vi "Project documentation.vi"(8 "error in":errorcluster, 10 "Theme":bool, 11 "Project in":refnum<vi>) -> (0 "error out":errorcluster)   [LabVIEW 2019, in "Panther Dashboard.lvlib"]
uses:
  Panther Dashboard.lvlib
panel:
  in  "Cancel":bool
  in  "Save":bool
  in  "Project Description":string
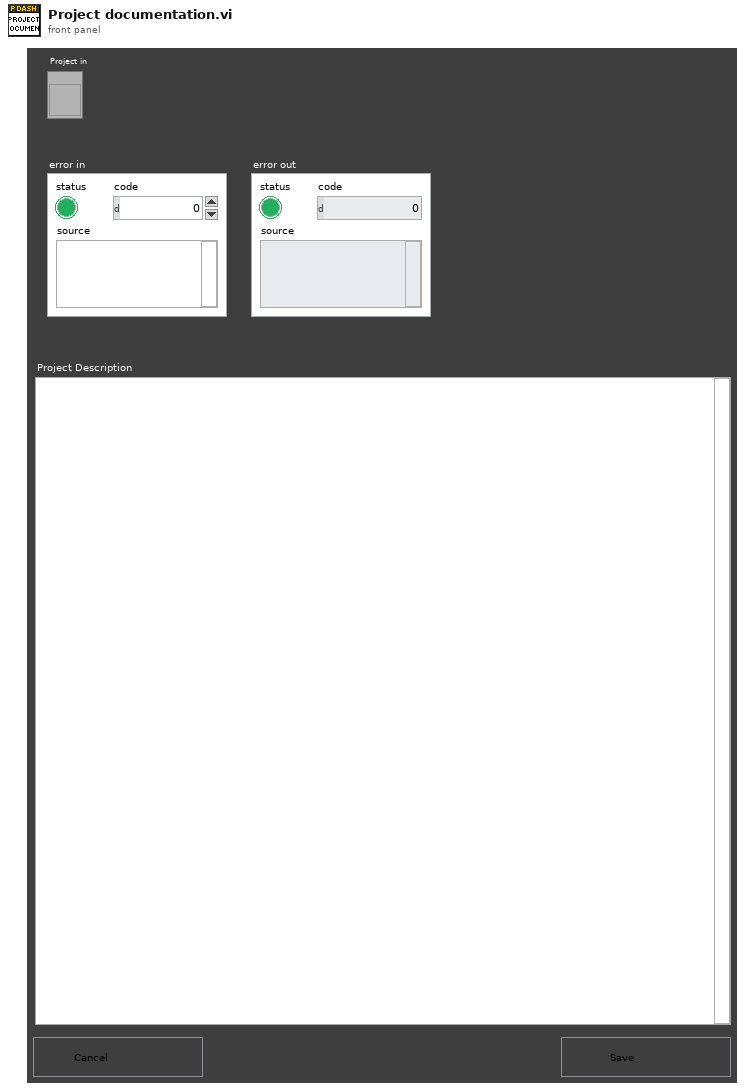
[diagram p1: front panel]
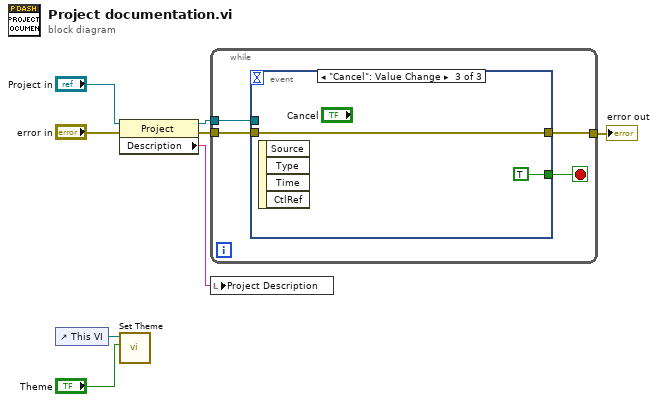
[diagram p0: block diagram]
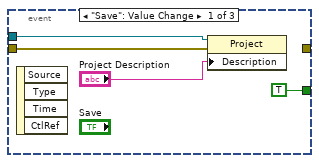
[diagram p2: hidden frame]
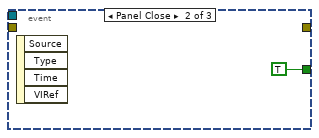
[diagram p3: hidden frame]
diagram:
  n1 = control-ref of="This VI"() -> (w3:refnum<vi>)
  n2 = property class="Project"(reference="Project in", error in="error in") -> (reference out=w4:refnum<vi>, error out=w7:errorcluster, "Description"=w5:string)
  n3 = call "Set Theme.vi"("Dark?"="Theme", "VI in"=w3) -> ()  [unwired: 10 in]
  n4 = while {
    tunnel: w7 -> [w12]
    tunnel: w4 -> [w11]
    tunnel: [w9] -> w1
    stop <- w10 stop-if-true
    n5 = event shown="[2] \"Cancel\": Value Change" {
      selector: _ -> [_ _ _]
      dyn-events: _ -> [_ _ _]
      timeout: _ -> [_ _ _]
      tunnel: w11 -> [w14 _ _]
      tunnel: w12 -> [w16 _ w18]
      tunnel: [TRUE TRUE TRUE] -> w10
      tunnel: [_ _ w18] -> w9
      event "Save": Value Change {
        n6 = event-data() -> ()  [unwired: 1 in, 4 out]
        n7 = property class="Project"(reference=w14, error in=w16, "Description"="Project Description") -> ()  [unwired: 2 out]
      }
      event Panel Close {
        n8 = event-data() -> ()  [unwired: 1 in, 4 out]
      }
      event "Cancel": Value Change {
        n9 = event-data() -> ()  [unwired: 1 in, 4 out]
      }
    }
  }
  "error out" <- w1
  n10 = local write "Project Description"(w5) -> ()
